vi "Narysowanie przesuniętej mapy.vi"(10 "Przesunięcie mapy":cluster{"X":i16, "Y":i16}, 11 "Mapa":picture) -> (3 "Przesunięta mapa":picture)   [LabVIEW 2012, in "Biblioteka moduł map v3.lvlib" / "Obsługa grafiki mapy.lvlib"]
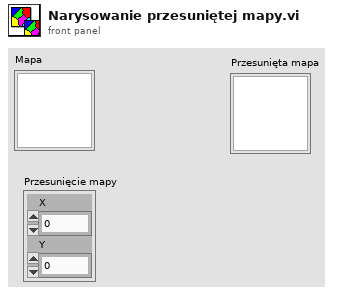
[diagram p1: front panel]
types:
  T1 = typedef "imagedata.ctl" = cluster{"image type":i32, "image depth":i32, "image":u8[], "mask":u8[], "colors":u32[], "Rectangle":cluster{"left":i16, "top":i16, "right":i16, "bottom":i16}}
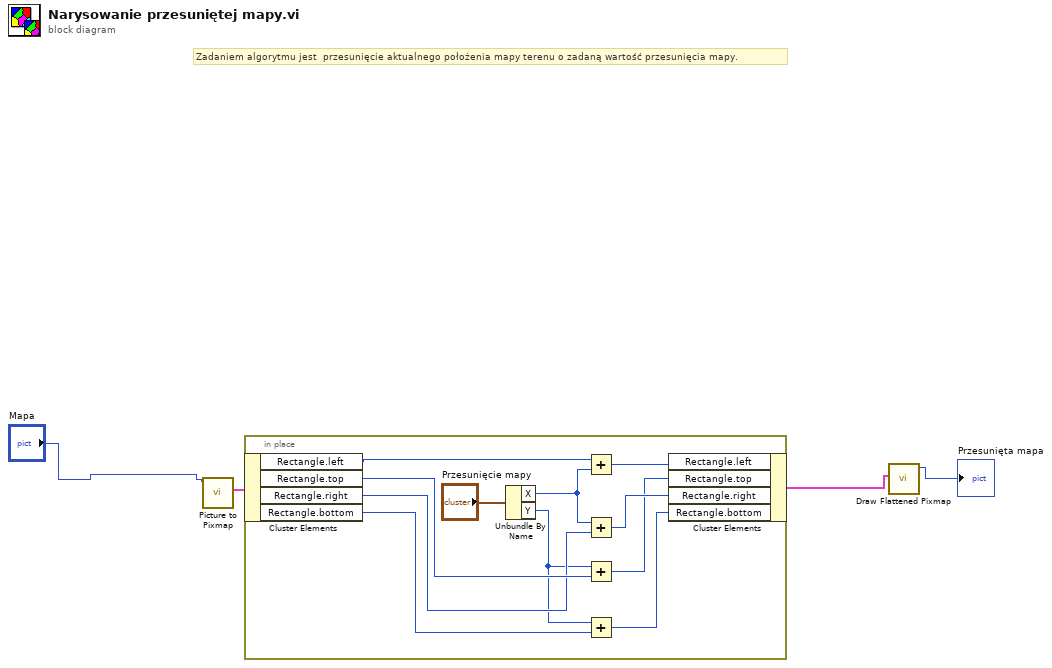
[diagram p0: block diagram]
diagram:
  # "Zadaniem algorytmu jest  przesunięcie aktualnego położenia mapy terenu o zadaną wartość przesunięcia mapy."
  n1 = call <vilib>:"Picture to Pixmap.vi"("picture"="Mapa") -> ("image data"=w1:T1)  [unwired: 9 in, 1 out]
  n2 = in-place {
    n3 = in-place-cluster #1(w1) -> ("Rectangle.left"=w15:i16, "Rectangle.top"=w14:i16, "Rectangle.right"=w13:i16, "Rectangle.bottom"=w12:i16)
    n4 = Unbundle By Name("Przesunięcie mapy") -> ("X"=w6:i16, "Y"=w7:i16)
    n5 = Add(x=w15, y=w6) -> (x+y=w11:i16)
    n6 = Add(x=w6, y=w13) -> (x+y=w10:i16)
    n7 = Add(x=w7, y=w14) -> (x+y=w9:i16)
    n8 = Add(x=w7, y=w12) -> (x+y=w8:i16)
    n9 = in-place-cluster #1("Rectangle.left"=w11, "Rectangle.top"=w9, "Rectangle.right"=w10, "Rectangle.bottom"=w8) -> (w4:T1)
  }
  n10 = call <vilib>:"Draw Flattened Pixmap.vi"("image data"=w4) -> ("new picture"=→"Przesunięta mapa":picture)  [unwired: 8 in]
